vi "Periodic Tasks.vi"(8 "error in":errorcluster) -> ()   [LabVIEW 2017]
doc: "This VI runs in parallel to other tasks. It can contain as many user-defined periodic loops as you need. These can carry out PID or other sorts of timed response."
uses:
  <vilib>/Analysis/baseanly.llb/Mean (DBL).vi
  <vilib>/Rock Robotics/WPI/Utilities/WPI_GetSetVariantRefNum.vi
  Robot Global Data.vi
  <vilib>/Rock Robotics/Network Tables/NT Read Boolean.vi
  <vilib>/Rock Robotics/Network Tables/NT Write Number.vi
  <vilib>/Rock Robotics/Network Tables/NT Write Numeric Array.vi
  <vilib>/Analysis/NI_AALBase.lvlib
panel:
  out "Arrayval":dbl
  out "Accelerations":T1
  out "Joy Y":dbl(graph)
  out "Avg Y":dbl
  out "Mean":dbl(graph)
  out "Current Joy Y Value":dbl
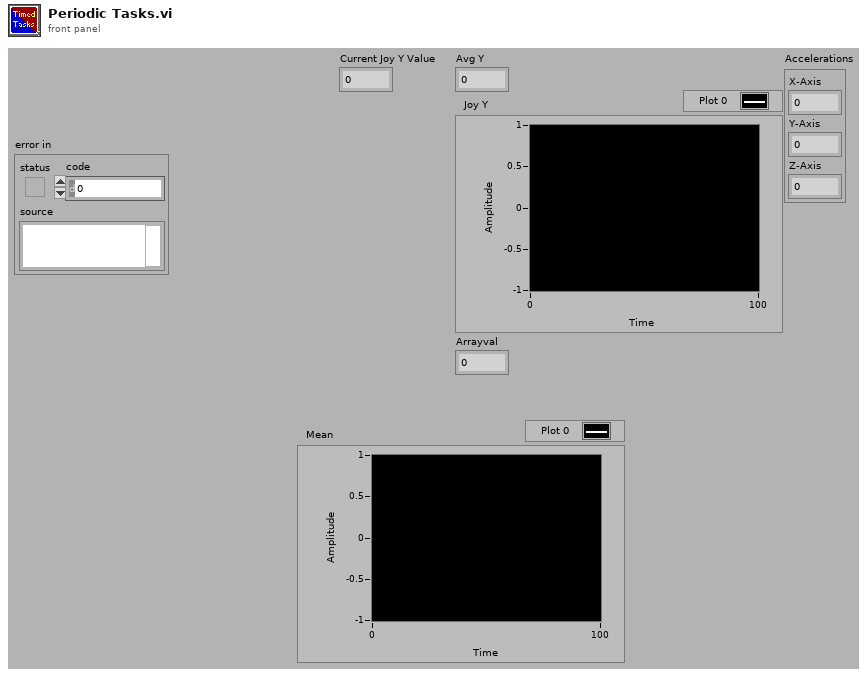
[diagram p1: front panel]
types:
  T1 = cluster{"X-Axis":dbl, "Y-Axis":dbl, "Z-Axis":dbl}
  T2 = typedef "WPI_JoystickDevRef.ctl" = cluster{"Device":T3}
  T3 = typedef "WPI_JoystickDeviceEnum.ctl" = enum16{"USB 0", "USB 1", "USB 2", "USB 3", "USB 4", "USB 5"}
  T4 = typedef "WPI_RobotDriveDevRef.ctl" = cluster{"DevStatus":errorcluster, "Motors[]":T5[], "Square Inputs":bool, "Max Output":dbl}
  T5 = typedef "WPI_MotorControlDeviceRef.ctl" = cluster{"DeviceStatus":errorcluster, "Type":T6, "PWM":cluster{"PWM Channel":T7, "DeadBand":T8}, "CAN":cluster{"Device Number":u8, "SetOutput VI Ref":variant, "GetOutput VI Ref":variant, "Enable VI Ref":variant, "Disable VI Ref":variant, "Data":variant}, "Invert":bool, "DIO PWM":cluster{"PWM \"Enable\" Channel":T7, "DIOChannel":T9, "PWM Rate":dbl}}
  T6 = typedef "WPI_MotorControlType.ctl" = enum16{"PWM", "CAN", "DIO PWM"}
  T7 = typedef "FPGA_DIOPWMChannel.ctl" = enum8{"PWM 0", "PWM 1", "PWM 2", "PWM 3", "PWM 4", "PWM 5", "PWM 6", "PWM 7", "PWM 8", "PWM 9", "PWM MXP 0", "PWM MXP 1", "PWM MXP 2", "PWM MXP 3", "PWM MXP 4", "PWM MXP 5", "PWM MXP 6", "PWM MXP 7", "PWM MXP 8", "PWM MXP 9", "Invalid"}
  T8 = typedef "WPI_PWMDeadband.ctl" = cluster{"Name":string, "maxPositivePwm":i32, "minPositivePwm":i32, "centerPwm":i32, "maxNegativePwm":i32, "minNegativePwm":i32, "angularRange":u16}
  T9 = typedef "FPGA_DIOChannel.ctl" = enum8{"DIO 0", "DIO 1", "DIO 2", "DIO 3", "DIO 4", "DIO 5", "DIO 6", "DIO 7", "DIO 8", "DIO 9", "DIO MXP 0", "DIO MXP 1", "DIO MXP 2", "DIO MXP 3", "DIO MXP 4", "DIO MXP 5", "DIO MXP 6", "DIO MXP 7", "DIO MXP 8", "DIO MXP 9", "DIO MXP 10", "DIO MXP 11", "DIO MXP 12", "DIO MXP 13", "DIO MXP 14", "DIO MXP 15", "SPI Port CS1", "SPI Port CS2", "SPI Port CS3", "SPI Port MISO", "SPI Port MOSI", "Invalid"}
  T10 = typedef "WPI_AccelerometerDevRef.ctl" = cluster{"DevStatus":errorcluster, "Scaling":T11, "Analog Channels":T12, "I2C Bus":T14, "SPI Bus":T15, "Accel Range":T16, "ADXL Axes":T17, "Handle":i32, "Device Address":u8, "Accel Type":enum16{"Analog", "ADXL345 I2C", "ADXL345 SPI", "Internal", "ADXL362 SPI"}}
  T11 = typedef "WPI_AccelerometerScaling.ctl" = cluster{"Gain (VoltsPerG)":dbl, "Center Voltage":dbl}
  T12 = typedef "WPI_AccelerometerAnalogChannels.ctl" = cluster{"X-Axis":T13, "Y-Axis":T13, "Z-Axis":T13}
  T13 = typedef "FPGA_AIChannel.ctl" = enum8{"AI 0", "AI 1", "AI 2", "AI 3", "AI MXP 0", "AI MXP 1", "AI MXP 2", "AI MXP 3", "Invalid"}
  T14 = typedef "i2c_bus.ctl" = enum16{"I2C On-Board", "I2C MXP", "Invalid"}
  T15 = typedef "spi_bus.ctl" = enum16{"SPI On-Board, CS0", "SPI On-Board, CS1", "SPI On-Board, CS2", "SPI On-Board, CS3", "SPI MXP", "Invalid"}
  T16 = typedef "ADXL345 Range.ctl" = u8
  T17 = typedef "WPI_AccelerometerADXL345 Axes.ctl" = cluster{"X-Axis":bool, "Y-Axis":bool, "Z-Axis":bool}
  T18 = typedef "WPI_GyroDevRef.ctl" = cluster{"DevStatus":errorcluster, "Analog Channel":T13, "Gain (VoltsPerDegree/Second)":dbl, "Gyro Type":enum16{"Analog", "XRS450"}, "Handle":i32, "SPI Bus":T15, "Device Found":bool, "Sample Rate":dbl, "Calibrate On Open":bool, "Offset":dbl}
  T19 = cluster{"JoystickDevRef":T2, "RobotDriveDevRef":T4}
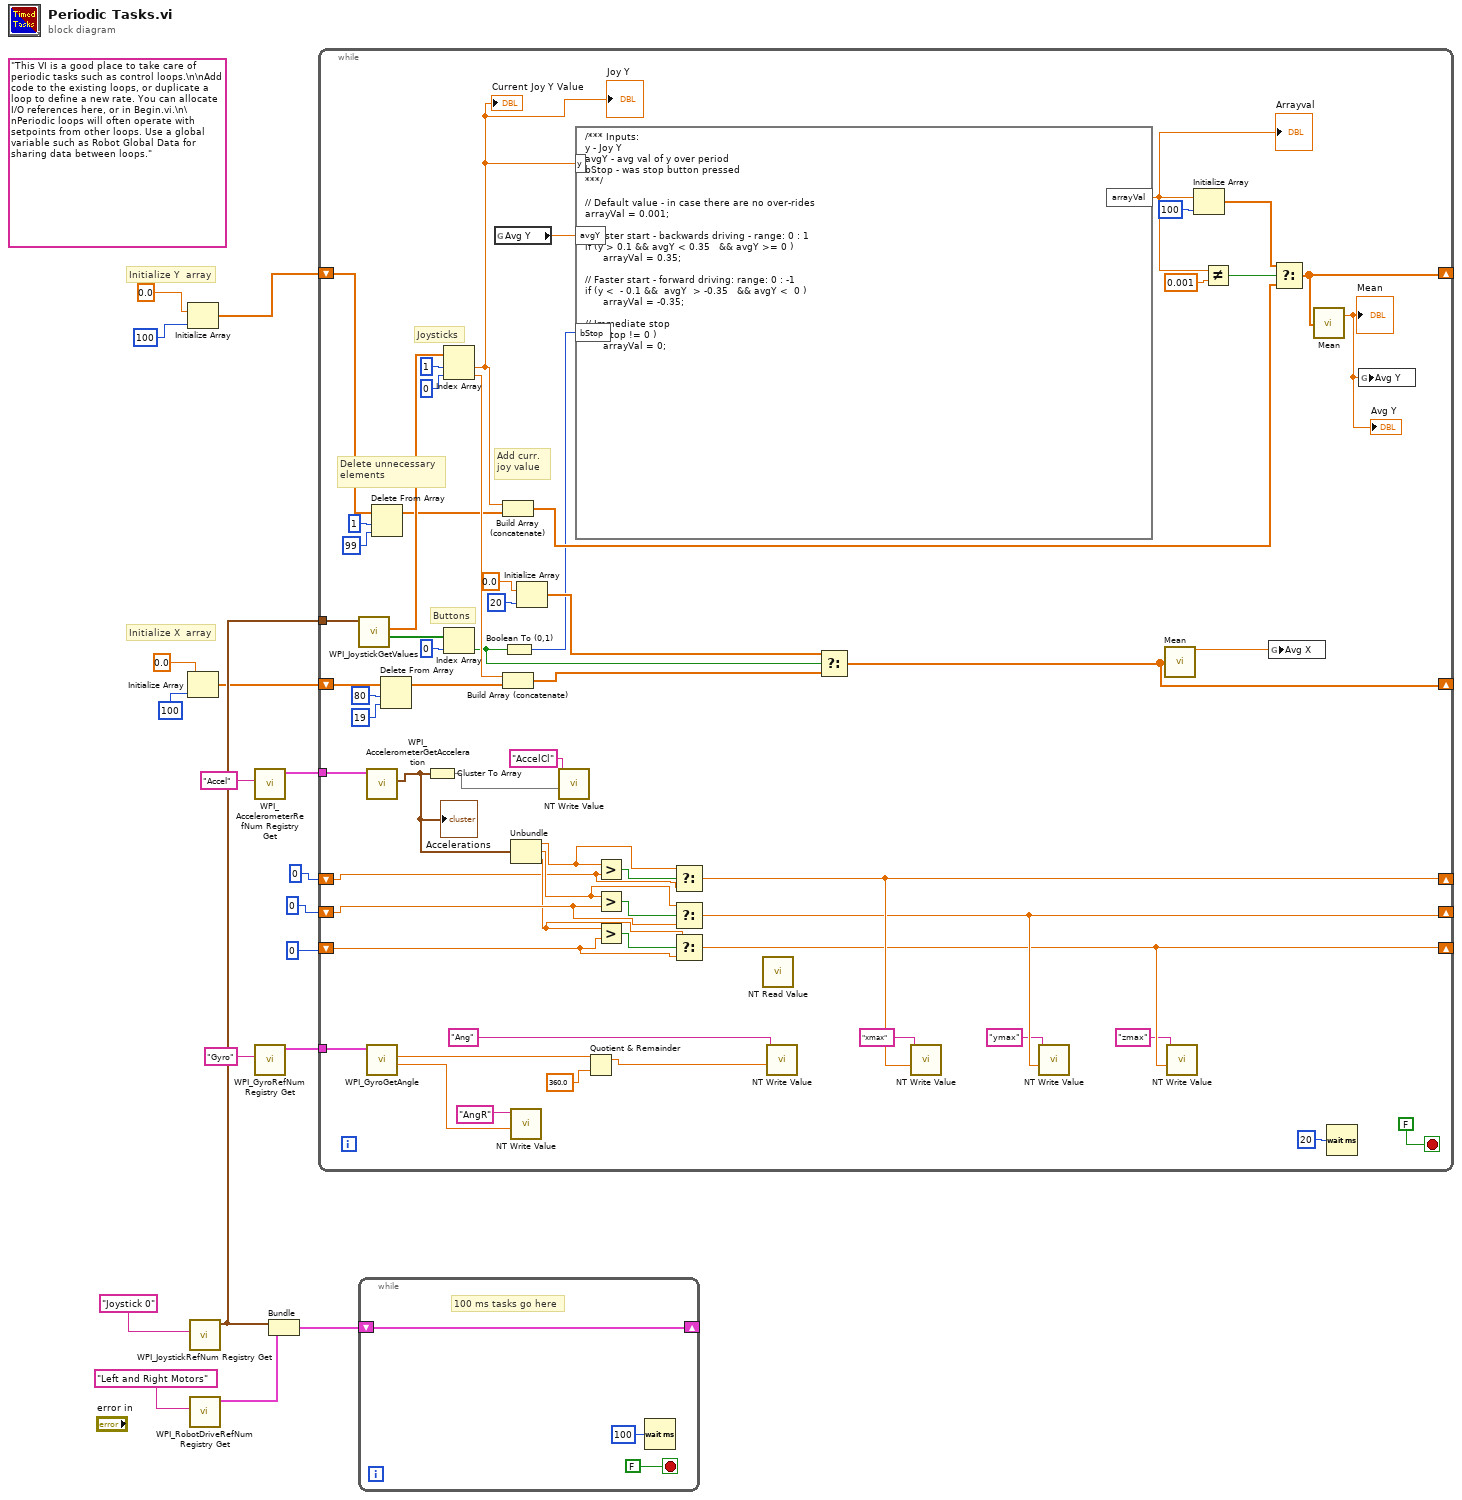
[diagram p0: block diagram]
diagram:
  (unwired) "This VI is a good place to take care of periodic tasks such as control loops.\n\nAdd code to the existing loops, or duplicate a loop to define a new rate. You can allocate I/O references here, or in Begin.vi.\n\nPeriodic loops will often operate with setpoints from other loops. Use a global variable such as Robot Global Data for sharing data between loops."
  # "Initialize X  array"
  # "Initialize Y  array"
  n1 = Initialize Array(0.0 ("element"), 100 ("dimension size")) -> (w11:dbl[])
  n2 = Initialize Array(0.0 ("element"), 100 ("dimension size")) -> (w10:dbl[])
  n3 = call <vilib>:"WPI_JoystickRefNum Registry Get.vi"("refnum name"="Joystick 0") -> ("JoystickDevRef"=w14:T2)  [unwired: 1 in, 9 out]
  n4 = call <vilib>:"WPI_RobotDriveRefNum Registry Get.vi"("refnum name"="Left and Right Motors") -> ("RobotDriveDevRef"=w16:T4)  [unwired: 1 in, 9 out]
  n5 = call <vilib>:"WPI_AccelerometerRefNum Registry Get.vi"("refnum name"="Accel") -> ("AccelerometerDevRef"=w6:T10)  [unwired: 9 in, 1 out]
  n6 = call <vilib>:"WPI_GyroRefNum Registry Get.vi"("refnum name"="Gyro") -> ("GyroDevRef"=w4:T18)  [unwired: 9 in, 1 out]
  n7 = Bundle("JoystickDevRef"=w14, "RobotDriveDevRef"=w16) -> (w15:T19)  [unwired: 1 out]
  n8 = while {
    tunnel: w14 -> [w77]
    shift-right: [w51] -> _
    shift-left: w11 -> [w74]
    shift-right: [w70] -> _
    shift-left: w10 -> [w64]
    tunnel: w6 -> [w46]
    tunnel: w4 -> [w45]
    shift-right: [w26] -> _
    shift-left: 0 -> [w27]
    shift-right: [w25] -> _
    shift-left: 0 -> [w30]
    shift-right: [w24] -> _
    shift-left: 0 -> [w28]
    stop <- FALSE stop-if-true
    # "Add curr. \njoy value"
    # "Delete unnecessary \nelements"
    # "Joysticks"
    # "Buttons"
    n9 = call <vilib>:"WPI_JoystickGetValues.vi"("JoystickDevRef"=w77) -> ("Buttons"=w73:bool[], "Axes"=w76:dbl[])  [unwired: 6 in, 3 out]
    n10 = call <vilib>:"WPI_AccelerometerGetAcceleration.vi"("AccelerometerDevRef"=w46) -> ("Accelerations"=w36:T1)  [unwired: 8 in, 2 out]
    "Accelerations" <- w36
    n11 = call <vilib>:"WPI_GyroGetAngle.vi"("GyroDevRef"=w45) -> ("Angular Rate"=w43:dbl, "Angle"=w38:dbl)  [unwired: 6 in, 3 out]
    n12 = Delete From Array(array=w74, length=1, index=99) -> (array with subset deleted=w56:dbl[])  [unwired: 1 out]
    n13 = Delete From Array(array=w64, length=80, index=19) -> (array with subset deleted=w66:dbl[])  [unwired: 1 out]
    n14 = Cluster To Array(cluster=w36) -> (array=w44:dbl[])
    n15 = Index Array(array=w76, index #1=1 ("index"), index #2=0 ("index")) -> (element #1=w47:dbl, element #2=w62:dbl)
    "Current Joy Y Value" <- w47
    "Joy Y" <- w47
    n16 = Index Array(array=w73, index=0) -> (element=w52:bool)
    n17 = global read "Robot Global Data.vi" "Avg Y"() -> (w54:dbl)
    n18 = Build Array (concatenate)(w47, w56) -> (w55:dbl[])
    n19 = Build Array (concatenate)(w62, w66) -> (w63:dbl[])
    n20 = Boolean To (0,1)(Boolean=w52) -> (0, 1=w53:i16)
    n21 = Unbundle(w36) -> ("X-Axis"=w34:dbl, "Y-Axis"=w31:dbl, "Z-Axis"=w29:dbl)
    n22 = call-poly <vilib>:"NT Write Value.vi"("Numeric"=w43, "Name"="AngR") -> ()  [unwired: 9 in, 1 out]
    n23 = Initialize Array(0.0 ("element"), 20 ("dimension size")) -> (w69:dbl[])
    n24 = call-poly <vilib>:"NT Write Value.vi"("Numeric Array"=w44, "Name"="AccelCl") -> ()  [unwired: 9 in, 1 out]
    n25 = formula code="/*** Inputs:\ny - Joy Y\navgY - avg val of y over period\nbStop - was stop button pressed\n***/\n\n// Default value - in case there are no over-rides\narrayVal = 0.001;\n\n// Faster start - backwards driving - range: 0 : 1\nif (y > 0.1 && avgY < 0.35   && avgY >= 0 )\n      arrayVal = 0.35;\n\n// Faster start - forward driving: range: 0 : -1\nif (y <  - 0.1 &&  avgY  > -0.35   && avgY <  0 )\n      arrayVal = -0.35;\n\n// Immediate stop\nif (bStop != 0 )\n      arrayVal = 0;"("y"=w47, "avgY"=w54, "bStop"=w53) -> ("arrayVal"=w48:dbl)
    "Arrayval" <- w48
    n26 = Quotient & Remainder(x=w38, y=360.0) -> (x-y*floor(x/y)=w37:dbl)  [unwired: 1 out]
    n27 = Greater?(x=w34, y=w27) -> (0:w35:bool)
    n28 = Greater?(x=w31, y=w30) -> (0:w33:bool)
    n29 = Greater?(x=w29, y=w28) -> (0:w32:bool)
    n30 = Select(t=w34, s=w35, f=w27) -> (s? t:f=w26:dbl)
    n31 = Select(t=w31, s=w33, f=w30) -> (s? t:f=w25:dbl)
    n32 = Select(t=w29, s=w32, f=w28) -> (s? t:f=w24:dbl)
    n33 = call-poly <vilib>:"NT Read Value.vi"() -> ()  [unwired: 10 in, 2 out]
    n34 = call-poly <vilib>:"NT Write Value.vi"("Numeric"=w37, "Name"="Ang") -> ()  [unwired: 9 in, 1 out]
    n35 = Select(t=w69, s=w52, f=w63) -> (s? t:f=w70:dbl[])
    n36 = call-poly <vilib>:"NT Write Value.vi"("Numeric"=w26, "Name"="xmax") -> ()  [unwired: 9 in, 1 out]
    n37 = call-poly <vilib>:"NT Write Value.vi"("Numeric"=w25, "Name"="ymax") -> ()  [unwired: 9 in, 1 out]
    n38 = call-poly <vilib>:"Mean.vi"("X"=w70) -> ("mean"=w20:dbl)  [unwired: 1 out]
    n39 = call-poly <vilib>:"NT Write Value.vi"("Numeric"=w24, "Name"="zmax") -> ()  [unwired: 9 in, 1 out]
    n40 = Initialize Array(w48, 100 ("dimension size")) -> (w58:dbl[])
    n41 = Not Equal?(x=w48, y=0.001) -> (x != y?=w50:bool)
    n42 = global write "Robot Global Data.vi" "Avg X"(w20) -> ()
    n43 = Select(t=w58, s=w50, f=w55) -> (s? t:f=w51:dbl[])
    n44 = call-poly <vilib>:"Mean.vi"("X"=w51) -> ("mean"=w19:dbl)  [unwired: 1 out]
    "Mean" <- w19
    "Avg Y" <- w19
    n45 = Wait (ms)(milliseconds to wait=u32 20) -> ()  [unwired: 1 out]
    n46 = global write "Robot Global Data.vi" "Avg Y"(w19) -> ()
  }
  n47 = while {
    shift-right: [w80] -> _
    shift-left: w15 -> [w80]
    stop <- FALSE stop-if-true
    # "100 ms tasks go here"
    n48 = Wait (ms)(milliseconds to wait=u32 100) -> ()  [unwired: 1 out]
  }
